vi "Get Helium Level.vi"(8 "error in (no error)":errorcluster, 11 "Instrument.Cryostat in":refnum<class "Instrument.Cryostat.lvclass">) -> (0 "error out":errorcluster, 2 "LHe Level (%)":dbl, 3 "Instrument.Cryostat out":refnum<class "Instrument.Cryostat.lvclass">)   [LabVIEW 2019, in "Instrument.Cryostat.lvclass"]
uses:
  Instrument.Cryostat.lvclass
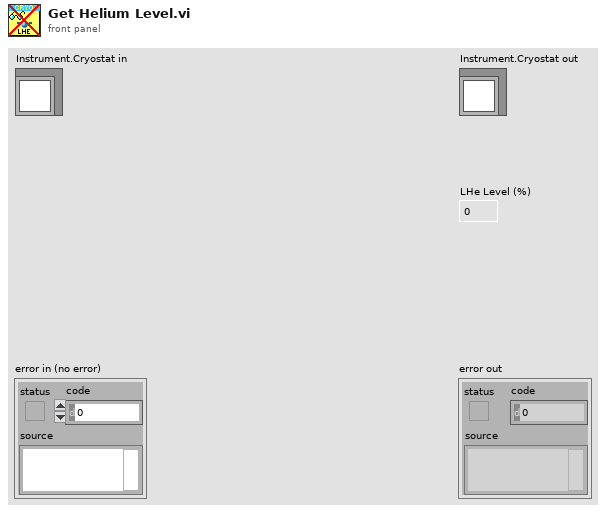
[diagram p1: front panel]
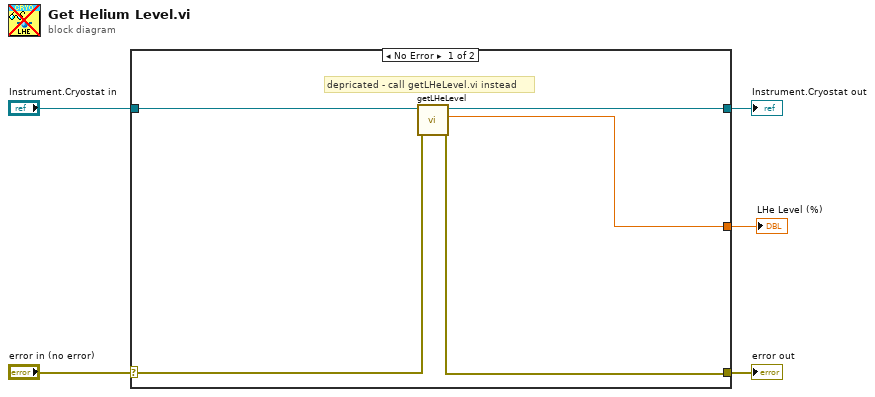
[diagram p0: block diagram]
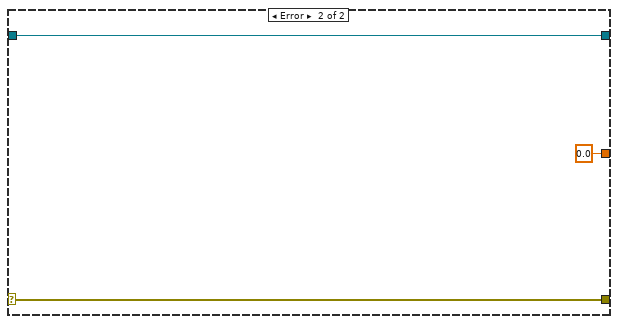
[diagram p2: hidden frame]
diagram:
  n1 = case shown="No Error" "error in (no error)" {
    selector: "error in (no error)" -> [w8 w13]
    tunnel: [w7 w13] -> w4
    tunnel: [w9 w12] -> w2
    tunnel: "Instrument.Cryostat in" -> [w10 w12]
    tunnel: [w6 0.0 ("LHe Level (%)")] -> w1
    frame No Error {
      # "depricated - call getLHeLevel.vi instead"
      n2 = call-dynamic "getLHeLevel.vi"("error in (no error)"=w8, "Instrument.Cryostat in"=w10) -> ("error out"=w7:errorcluster, "LHe Level (%)"=w6:dbl, "Instrument.Cryostat out"=w9:refnum<class "Instrument.Cryostat.lvclass">)  [unwired: 7 in]
    }
    frame Error {
    }
  }
  "error out" <- w4
  "Instrument.Cryostat out" <- w2
  "LHe Level (%)" <- w1
